vi "Camera_LocalYUV.vi"(0 "Location":cluster{"X":sgl, "Y":sgl}, 2 "SRV In":string) -> (1 "YUV":cluster{"Y":sgl, "U":sgl, "V":sgl}, 4 "SRV Out":string="169.254.0.10")   [LabVIEW 2009]
panel:
  out "data out":string
  # "This LabVIEW item is deprecated.\n\nIt is believed to be unused and will be removed in a future version of SRV."
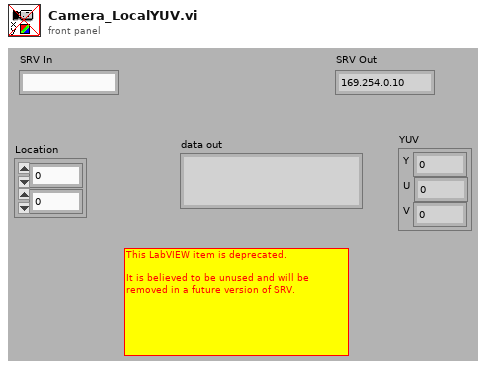
[diagram p1: front panel]
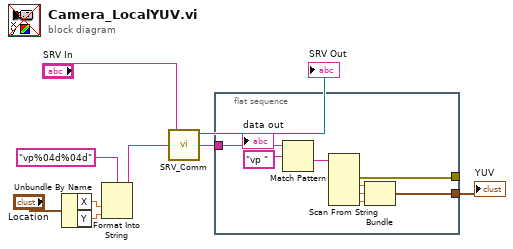
[diagram p0: block diagram]
diagram:
  n1 = Unbundle By Name("Location") -> ("X"=w2:sgl, "Y"=w1:sgl)
  n2 = Format Into String(format string="vp%04d%04d", w2, w1) -> (resulting string=w4:string)  [unwired: 2 in, 1 out]
  n3 = call "SRV_Comm.vi"("Command Sent"=w4, "SRV In"="SRV In") -> ("Reply"=w9:string, "SRV Out"=→"SRV Out":refnum<k5>)  [unwired: 1 in, 1 out]
  n4 = flat-sequence {
    tunnel: w9 -> [w17]
    tunnel: [w14] -> _
    tunnel: [w10] -> w6
    frame #0 {
      n5 = Match Pattern(string=w17, regular expression="vp " ("Command Sent")) -> (after substring=w16:string)  [unwired: 1 in, 3 out]
      n6 = Scan From String(input string=w16) -> (error out=w14:errorcluster, output 1=w11:dbl, output 2=w12:dbl, output 3=w13:dbl)  [unwired: 6 in, 2 out]
      n7 = Bundle(w11, w12, w13) -> (w10:cluster{dbl, dbl, dbl})  [unwired: 1 in]
      "data out" <- w17
    }
  }
  "YUV" <- w6
